vi "Get Sub Object.vi"(8 "error in":errorcluster, 10 "Sub Index":u8, 11 "Obj Entry in":refnum<class "Object Entry.lvclass">) -> (0 "error out":errorcluster, 1 "Sub Object":refnum<class "Sub Object.lvclass">, 3 "Obj Entry out":refnum<class "Object Entry.lvclass">)   [LabVIEW 2020, in "CANopen.lvlib" / "Object Entry.lvclass"]
doc: "This method combines the functionality of the Contains Sub Object method and the Get Sub Object. Use the Try Get Sub Object method if your code frequently attempts to access keys that are not in the dictionary. Using this method is more efficient than catching the Error from by the Get Sub Object method."
uses:
  Object Entry.lvclass
  Sub Object/Sub Object.lvclass
  Object Entry.lvclass/Object Entry.ctl
  Sub Objects Dictionary/Sub Objects Dictionary.lvclass
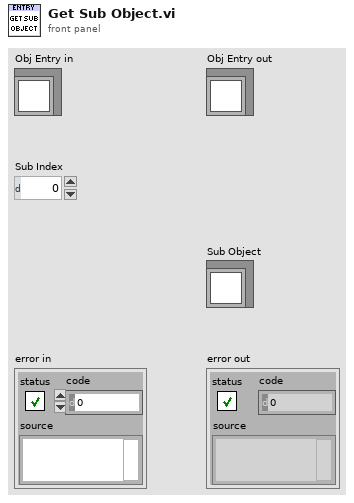
[diagram p1: front panel]
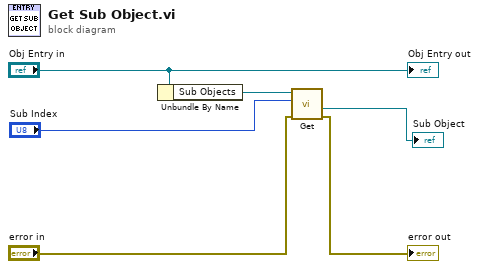
[diagram p0: block diagram]
diagram:
  n1 = Unbundle By Name("Obj Entry in") -> ("Sub Objects"=w2:refnum<class "Sub Objects Dictionary.lvclass">)
  n2 = call "Get.vi"("error in"="error in", "Sub Index"="Sub Index", "Sub Objects Dictionary in"=w2) -> ("error out"=→"error out":errorcluster, "Sub Obj"=→"Sub Object":refnum<class "Sub Object.lvclass">)  [unwired: 6 in, 1 out]
  "Obj Entry out" <- "Obj Entry in"
